vi "SDCP SMF Rx Logger - FGV (version 1.0).vi"(2 "error in (no error)":errorcluster, 3 "Commands":T2) -> (0 "error out":errorcluster, 1 "Rx data":T1[](array[typedef]))   [LabVIEW 2020]
uses:
  SDCP SMF Rx Logger - FGV - Commands.vi
  Typedefs/SDCP SMF logger - SMF with timestamp.ctl
  Typedefs/SDCP SMF Rx Logger - Notifier FGV - Notifier names.ctl
  Typedefs/SDCP SMF Rx Logger - Notifier FGV - Commands.ctl
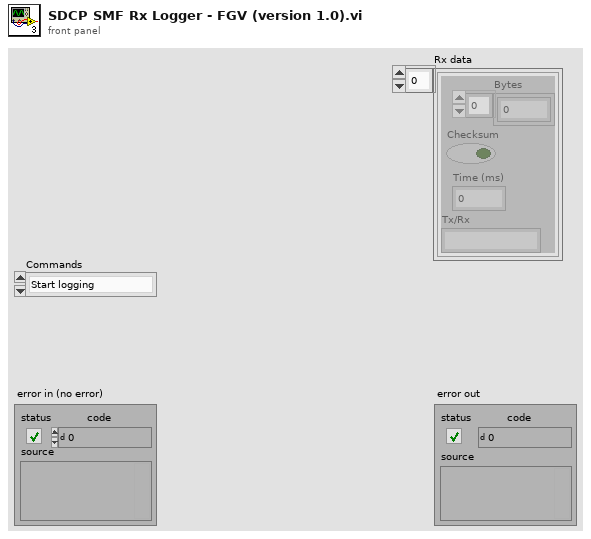
[diagram p1: front panel]
types:
  T1 = typedef "SDCP SMF logger - SMF with timestamp.ctl" = cluster{"Bytes":u8[], "Checksum":bool, "Time (ms)":u32, "Tx/Rx":string}
  T2 = typedef "SDCP SMF Rx Logger - FGV - Commands.vi" = enum16{"Start logging", "Pause logging", "Get log data", "Reset log", "Stop logging"}
  T3 = typedef "SDCP SMF Rx Logger - Notifier FGV - Commands.ctl" = enum16{"Initialize", "Read", "Write", "Deinitialize"}
  T4 = typedef "SDCP SMF Rx Logger - Notifier FGV - Notifier names.ctl" = enum16{"Logged data", "Pause logging", "Get log", "Reset log", "Sample counter", "Logged data buffer", "Stop logging"}
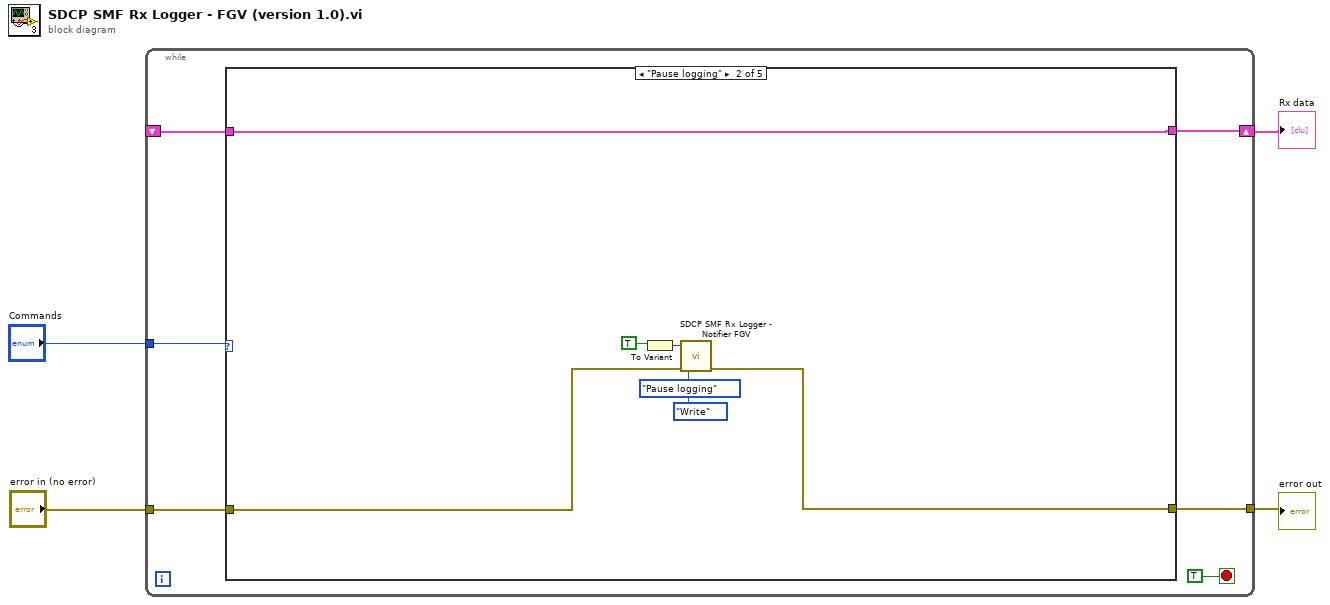
[diagram p0: block diagram]
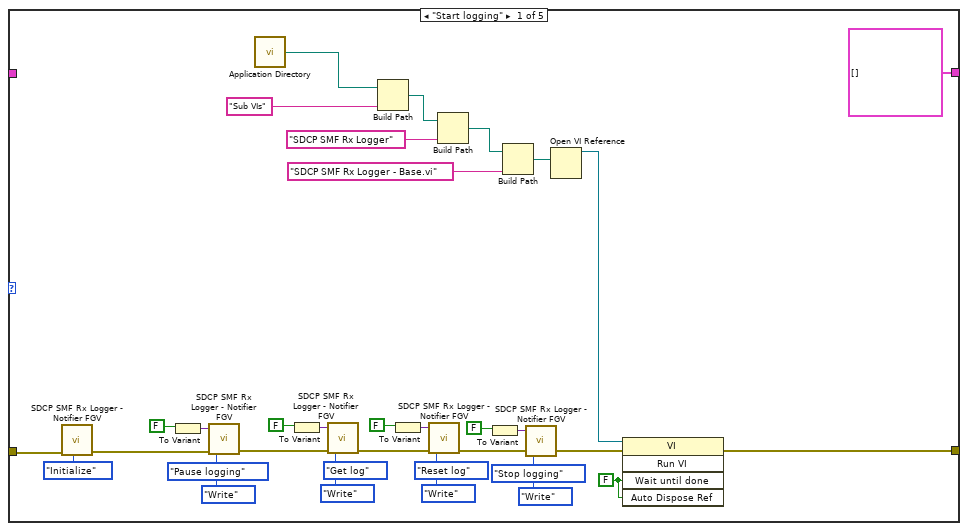
[diagram p2: hidden frame]
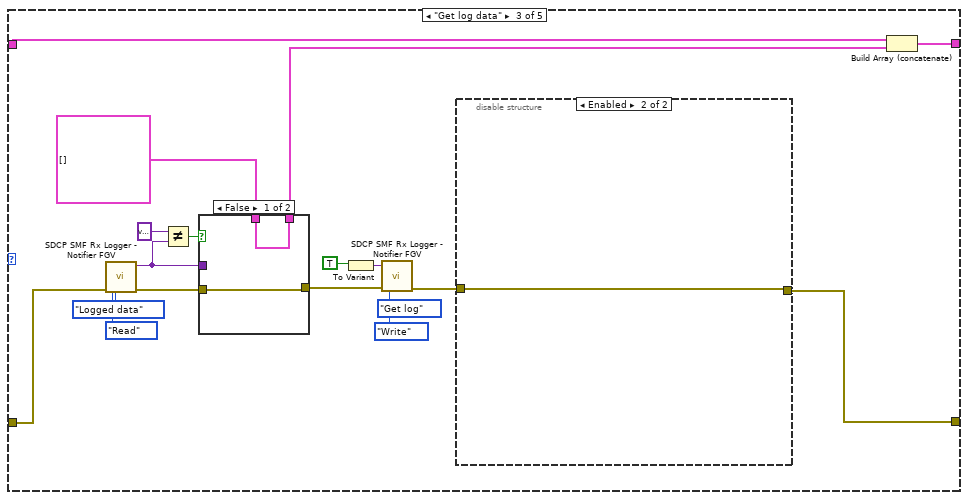
[diagram p3: hidden frame]
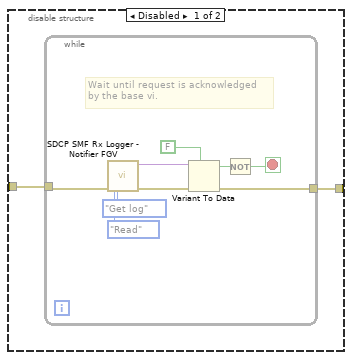
[diagram p4: hidden frame]
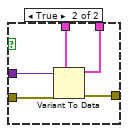
[diagram p5: hidden frame]
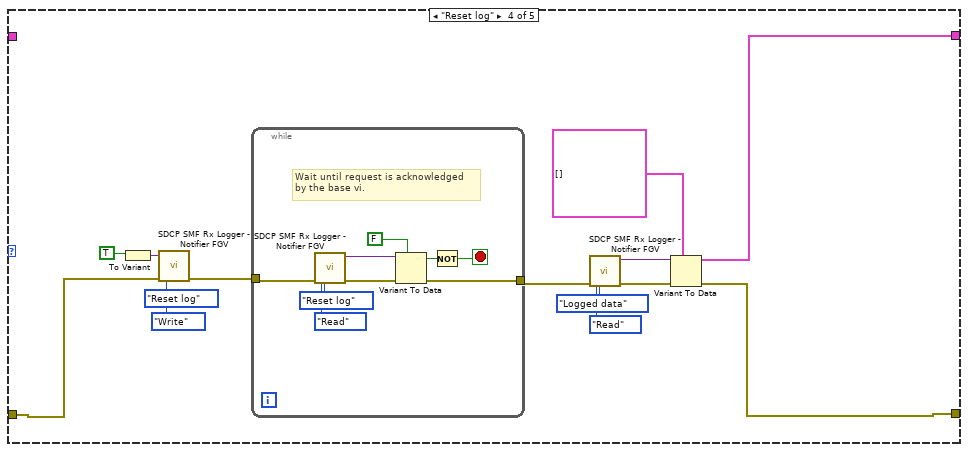
[diagram p6: hidden frame]
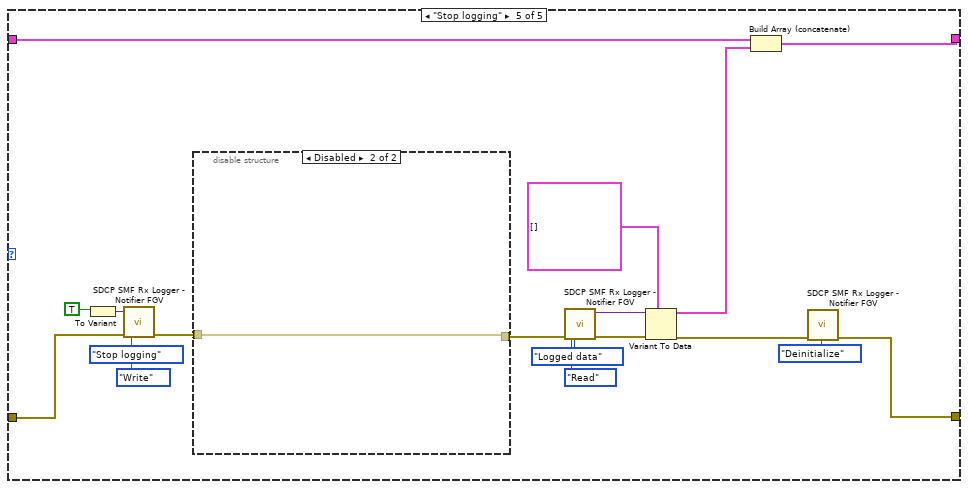
[diagram p7: hidden frame]
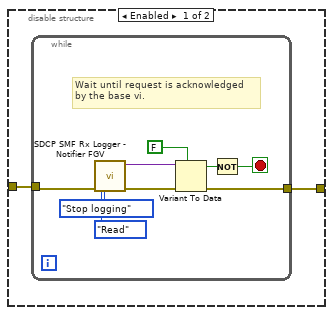
[diagram p8: hidden frame]
diagram:
  n1 = while {
    tunnel: "error in (no error)" -> [w8]
    tunnel: "Commands" -> [w9]
    tunnel: [w7] -> w2
    shift-right: [w5] -> w1
    shift-left: _ -> [w6]
    stop <- TRUE stop-if-true
    n2 = case shown="\"Pause logging\"" w9 {
      tunnel: w8 -> [w44 w47 w58 w91 w124]
      tunnel: [w15 w46 w57 w90 w112] -> w7
      tunnel: w6 -> [_ w45 w59 _ w117]
      tunnel: [T1[] [] w45 w60 w89 w115] -> w5
      frame "Start logging" {
        w16 = FALSE ("Wait Until Done")
        n3 = call "SDCP SMF Rx Logger - Notifier FGV.vi"("error in (no error)"=w44, "Command"=SDCP_SMF_Rx_Logger_-_Notifier_FGV_-_Commands."Initialize") -> ("error out"=w42:errorcluster)  [unwired: 4 in, 1 out]
        n4 = To Variant(anything=FALSE) -> (Variant=w39:variant)
        n5 = call "SDCP SMF Rx Logger - Notifier FGV.vi"("error in (no error)"=w42, "Command"=SDCP_SMF_Rx_Logger_-_Notifier_FGV_-_Commands."Write", "Notifier name"=SDCP_SMF_Rx_Logger_-_Notifier_FGV_-_Notifier_names."Pause logging", "Notifier value in"=w39) -> ("error out"=w33:errorcluster)  [unwired: 2 in, 1 out]
        n6 = call <vilib>:"Application Directory.vi"() -> ("Application Directory"=w11:path)
        n7 = To Variant(anything=FALSE) -> (Variant=w35:variant)
        n8 = call "SDCP SMF Rx Logger - Notifier FGV.vi"("error in (no error)"=w33, "Command"=SDCP_SMF_Rx_Logger_-_Notifier_FGV_-_Commands."Write", "Notifier name"=SDCP_SMF_Rx_Logger_-_Notifier_FGV_-_Notifier_names."Get log", "Notifier value in"=w35) -> ("error out"=w28:errorcluster)  [unwired: 2 in, 1 out]
        n9 = Build Path(base path=w11, name or relative path="Sub VIs") -> (appended path=w12:path)
        n10 = To Variant(anything=FALSE) -> (Variant=w30:variant)
        n11 = call "SDCP SMF Rx Logger - Notifier FGV.vi"("error in (no error)"=w28, "Command"=SDCP_SMF_Rx_Logger_-_Notifier_FGV_-_Commands."Write", "Notifier name"=SDCP_SMF_Rx_Logger_-_Notifier_FGV_-_Notifier_names."Reset log", "Notifier value in"=w30) -> ("error out"=w23:errorcluster)  [unwired: 2 in, 1 out]
        n12 = Build Path(base path=w12, name or relative path="SDCP SMF Rx Logger") -> (appended path=w21:path)
        n13 = To Variant(anything=FALSE) -> (Variant=w25:variant)
        n14 = Build Path(base path=w21, name or relative path="SDCP SMF Rx Logger - Base.vi") -> (appended path=w19:path)
        n15 = call "SDCP SMF Rx Logger - Notifier FGV.vi"("error in (no error)"=w23, "Command"=SDCP_SMF_Rx_Logger_-_Notifier_FGV_-_Commands."Write", "Notifier name"=SDCP_SMF_Rx_Logger_-_Notifier_FGV_-_Notifier_names."Stop logging", "Notifier value in"=w25) -> ("error out"=w18:errorcluster)  [unwired: 2 in, 1 out]
        n16 = Open VI Reference(vi path=w19) -> (vi reference=w17:refnum<vi>)  [unwired: 5 in, 1 out]
        n17 = invoke class="VI" method="Run VI"(reference=w17, error in=w18, "Wait until done"=w16, "Auto Dispose Ref"=w16) -> (error out=w15:errorcluster)  [unwired: 1 in, 4 out]
      }
      frame "Pause logging" {
        n18 = To Variant(anything=TRUE) -> (Variant=w49:variant)
        n19 = call "SDCP SMF Rx Logger - Notifier FGV.vi"("error in (no error)"=w47, "Command"=SDCP_SMF_Rx_Logger_-_Notifier_FGV_-_Commands."Write", "Notifier name"=SDCP_SMF_Rx_Logger_-_Notifier_FGV_-_Notifier_names."Pause logging", "Notifier value in"=w49) -> ("error out"=w46:errorcluster)  [unwired: 2 in, 1 out]
      }
      frame "Get log data" {
        n20 = call "SDCP SMF Rx Logger - Notifier FGV.vi"("error in (no error)"=w58, "Command"=SDCP_SMF_Rx_Logger_-_Notifier_FGV_-_Commands."Read", "Notifier name"=SDCP_SMF_Rx_Logger_-_Notifier_FGV_-_Notifier_names."Logged data") -> ("error out"=w62:errorcluster, "Notifier value out"=w54:variant)  [unwired: 3 in]
        n21 = Not Equal?(x=variant, y=w54) -> (x != y?=w55:bool)
        n22 = case shown="False" w55 {
          tunnel: w62 -> [w83 w88]
          tunnel: w54 -> [_ w87]
          tunnel: T1[] [] -> [w82 w86]
          tunnel: [w83 w85] -> w56
          tunnel: [w82 w84] -> w52
          frame False {
          }
          frame True {
            n23 = Variant To Data(error in=w88, type=w86, Variant=w87) -> (data=w84:T1[], error out=w85:errorcluster)
          }
        }
        n24 = To Variant(anything=TRUE) -> (Variant=w67:variant)
        n25 = call "SDCP SMF Rx Logger - Notifier FGV.vi"("error in (no error)"=w56, "Command"=SDCP_SMF_Rx_Logger_-_Notifier_FGV_-_Commands."Write", "Notifier name"=SDCP_SMF_Rx_Logger_-_Notifier_FGV_-_Notifier_names."Get log", "Notifier value in"=w67) -> ("error out"=w65:errorcluster)  [unwired: 2 in, 1 out]
        n26 = disable-structure shown="Enabled" {
          disable-tunnel: w65 -> [w71 w81]
          disable-tunnel: [w70 w81] -> w57
          frame Disabled {
            n27 = while {
              tunnel: w71 -> [w80]
              tunnel: [w72] -> w70
              stop <- w73 stop-if-true
              # "Wait until request is acknowledged\nby the base vi."
              n28 = call "SDCP SMF Rx Logger - Notifier FGV.vi"("error in (no error)"=w80, "Command"=SDCP_SMF_Rx_Logger_-_Notifier_FGV_-_Commands."Read", "Notifier name"=SDCP_SMF_Rx_Logger_-_Notifier_FGV_-_Notifier_names."Get log") -> ("error out"=w77:errorcluster, "Notifier value out"=w75:variant)  [unwired: 3 in]
              n29 = Variant To Data(error in=w77, type=FALSE, Variant=w75) -> (data=w74:bool, error out=w72:errorcluster)
              n30 = Not(x=w74) -> (.not. x?=w73:bool)
            }
          }
          frame Enabled {
          }
        }
        n31 = Build Array (concatenate)(w59, w52) -> (w60:T1[])
      }
      frame "Reset log" {
        n32 = To Variant(anything=TRUE) -> (Variant=w100:variant)
        n33 = call "SDCP SMF Rx Logger - Notifier FGV.vi"("error in (no error)"=w91, "Command"=SDCP_SMF_Rx_Logger_-_Notifier_FGV_-_Commands."Write", "Notifier name"=SDCP_SMF_Rx_Logger_-_Notifier_FGV_-_Notifier_names."Reset log", "Notifier value in"=w100) -> ("error out"=w98:errorcluster)  [unwired: 2 in, 1 out]
        n34 = while {
          tunnel: w98 -> [w111]
          tunnel: [w103] -> w93
          stop <- w104 stop-if-true
          # "Wait until request is acknowledged\nby the base vi."
          n35 = call "SDCP SMF Rx Logger - Notifier FGV.vi"("error in (no error)"=w111, "Command"=SDCP_SMF_Rx_Logger_-_Notifier_FGV_-_Commands."Read", "Notifier name"=SDCP_SMF_Rx_Logger_-_Notifier_FGV_-_Notifier_names."Reset log") -> ("error out"=w108:errorcluster, "Notifier value out"=w106:variant)  [unwired: 3 in]
          n36 = Variant To Data(error in=w108, type=FALSE, Variant=w106) -> (data=w105:bool, error out=w103:errorcluster)
          n37 = Not(x=w105) -> (.not. x?=w104:bool)
        }
        n38 = call "SDCP SMF Rx Logger - Notifier FGV.vi"("error in (no error)"=w93, "Command"=SDCP_SMF_Rx_Logger_-_Notifier_FGV_-_Commands."Read", "Notifier name"=SDCP_SMF_Rx_Logger_-_Notifier_FGV_-_Notifier_names."Logged data") -> ("error out"=w95:errorcluster, "Notifier value out"=w94:variant)  [unwired: 3 in]
        n39 = Variant To Data(error in=w95, type=T1[] [], Variant=w94) -> (data=w89:T1[], error out=w90:errorcluster)
      }
      frame "Stop logging" {
        n40 = To Variant(anything=TRUE) -> (Variant=w127:variant)
        n41 = call "SDCP SMF Rx Logger - Notifier FGV.vi"("error in (no error)"=w124, "Command"=SDCP_SMF_Rx_Logger_-_Notifier_FGV_-_Commands."Write", "Notifier name"=SDCP_SMF_Rx_Logger_-_Notifier_FGV_-_Notifier_names."Stop logging", "Notifier value in"=w127) -> ("error out"=w125:errorcluster)  [unwired: 2 in, 1 out]
        n42 = disable-structure shown="Disabled" {
          disable-tunnel: w125 -> [w131 w141]
          disable-tunnel: [w130 w141] -> w118
          frame Enabled {
            n43 = while {
              tunnel: w131 -> [w140]
              tunnel: [w132] -> w130
              stop <- w133 stop-if-true
              # "Wait until request is acknowledged\nby the base vi."
              n44 = call "SDCP SMF Rx Logger - Notifier FGV.vi"("error in (no error)"=w140, "Command"=SDCP_SMF_Rx_Logger_-_Notifier_FGV_-_Commands."Read", "Notifier name"=SDCP_SMF_Rx_Logger_-_Notifier_FGV_-_Notifier_names."Stop logging") -> ("error out"=w137:errorcluster, "Notifier value out"=w135:variant)  [unwired: 3 in]
              n45 = Variant To Data(error in=w137, type=FALSE, Variant=w135) -> (data=w134:bool, error out=w132:errorcluster)
              n46 = Not(x=w134) -> (.not. x?=w133:bool)
            }
          }
          frame Disabled {
          }
        }
        n47 = call "SDCP SMF Rx Logger - Notifier FGV.vi"("error in (no error)"=w118, "Command"=SDCP_SMF_Rx_Logger_-_Notifier_FGV_-_Commands."Read", "Notifier name"=SDCP_SMF_Rx_Logger_-_Notifier_FGV_-_Notifier_names."Logged data") -> ("error out"=w121:errorcluster, "Notifier value out"=w120:variant)  [unwired: 3 in]
        n48 = Variant To Data(error in=w121, type=T1[] [], Variant=w120) -> (data=w116:T1[], error out=w114:errorcluster)
        n49 = Build Array (concatenate)(w117, w116) -> (w115:T1[])
        n50 = call "SDCP SMF Rx Logger - Notifier FGV.vi"("error in (no error)"=w114, "Command"=SDCP_SMF_Rx_Logger_-_Notifier_FGV_-_Commands."Deinitialize") -> ("error out"=w112:errorcluster)  [unwired: 4 in, 1 out]
      }
    }
  }
  "error out" <- w2
  "Rx data" <- w1
